vi "Test Binning.vi"(11 "Test Case In":refnum<class "Test.Camera.lvclass">) -> (0 "error out":errorcluster, 3 "Test Case Out":refnum<class "Test.Camera.lvclass">)   [LabVIEW 2020, in "Test.Camera.lvclass"]
uses:
  Test.Camera.lvclass
  C:/Program Files (x86)/National Instruments/LabVIEW 2020/vi.lib/Astemes/LUnit/Test Case.lvclass
  g_industrial_cam/Camera/Camera.lvclass/Camera.ctl
  <vilib>/Astemes/LUnit/Test Case.lvclass/Test Case.ctl
  c3e2611f-c54f-4219-a549-b8da21c7f085.vi
  c7776276-95e4-4134-9906-b61dd734a09f.vi
  e74630cf-9c8b-4a3c-8b50-f04e46fa7099.vi
  0aa1576c-e916-4ad0-9a97-64bd3e4eb69b.vi
  g_industrial_cam/Camera/GetSetBinning.vi
  <vilib>/Astemes/LUnit/Core/LUnit Test Case/Private/Append Pass Result.vi
  <vilib>/Astemes/LUnit/Core/LUnit Test Case/Private/Append Fail Result.vi
  0aa1576c-e916-4ad0-9a97-64bd3e4eb69b.vi/9c5d11cd-9439-4240-a1ee-d9baace9c924.vi
  <vilib>/Astemes/LUnit/Core/LUnit Test Case/Private/Run In UI.vi
  <vilib>/Utility/error.llb/Clear Errors.vi
  g_industrial_cam/Camera/Check Not Disconnected.vi
  <vilib>/Utility/error.llb/Error Cluster From Error Code.vi
  Test.Camera.lvclass/Test.Camera.ctl
  <vilib>/Astemes/LUnit/Test Case.lvclass
  g_industrial_cam/Camera/Camera.lvclass
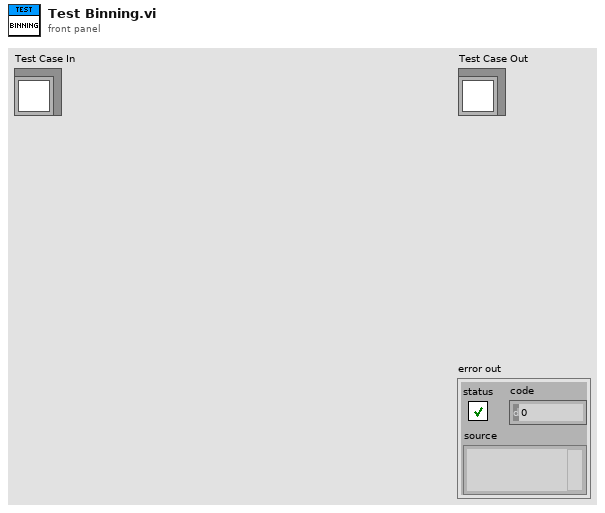
[diagram p1: front panel]
types:
  T1 = cluster{"dy Increment":i32, "dy Min":i32, "dy Max":i32, "dx Increment":i32, "dx Min":i32, "dx Max":i32, "dx":i32, "dy":i32, "Binning Avaliable":bool}
  T2 = cluster{"Alternative Value":i32, "Alternative Value":i32}
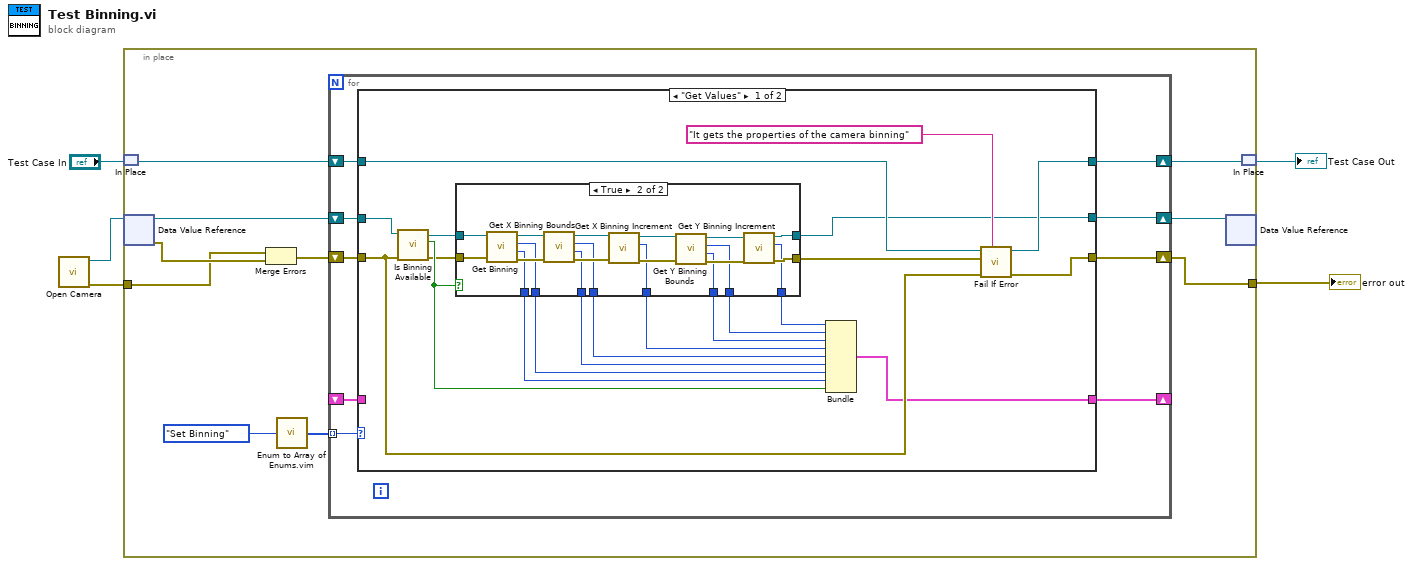
[diagram p0: block diagram]
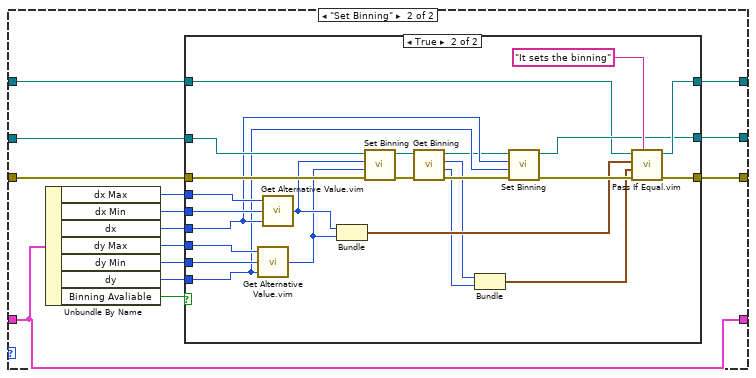
[diagram p3: hidden frame]
diagram:
  n1 = call "Open Camera.vi"() -> ("error out"=w5:errorcluster, "Camera"=w4:refnum<data-value>)  [unwired: 10 in]
  n2 = in-place {
    in-place-border: w5 -> [w9]
    in-place-border: [w8] -> w2
    n3 = in-place-match #1("Test Case In") -> (w10:refnum<class "Test.Camera.lvclass">)
    n4 = in-place-dvr #2(w4) -> (w14:refnum<class "Camera.lvclass">, w15:errorcluster)
    n5 = Merge Errors(w9, w15) -> (w13:errorcluster)
    n6 = call "Enum to Array of Enums.vim"("enum"=enum16{"Get Values", "Set Binning"}."Set Binning") -> ("array of enums"=w11:enum16{"Get Values", "Set Binning"}[])
    n7 = for {
      tunnel: w11 -> [w22] mode=indexing
      shift-right: [w21] -> w6
      shift-left: w14 -> [w24]
      shift-right: [w20] -> _
      shift-left: _ -> [w19]
      shift-right: [w17] -> w7
      shift-left: w10 -> [w18]
      shift-right: [w16] -> w8
      shift-left: w13 -> [w23]
      n8 = case shown="\"Get Values\"" w22 {
        tunnel: w24 -> [w40 w76]
        tunnel: w23 -> [w39 w77]
        tunnel: [w25 w69] -> w21
        tunnel: [w26 w78] -> w20
        tunnel: w19 -> [_ w78]
        tunnel: w18 -> [w44 w67]
        tunnel: [w43 w80] -> w17
        tunnel: [w41 w79] -> w16
        frame "Get Values" {
          n9 = call "Is Binning Available.vi"("error in (no error)"=w39, "Camera in"=w40) -> ("error out"=w37:errorcluster, "Binning Avaliable"=w38:bool, "Camera"=w36:refnum<class "Camera.lvclass">)  [unwired: 7 in]
          n10 = case shown="True" w38 {
            tunnel: w37 -> [w45 w66]
            tunnel: w36 -> [w46 w65]
            tunnel: [_ w59] -> w35
            tunnel: [_ w58] -> w34
            tunnel: [_ w57] -> w33
            tunnel: [_ w56] -> w32
            tunnel: [_ w55] -> w31
            tunnel: [_ w54] -> w30
            tunnel: [_ w53] -> w29
            tunnel: [w45 w52] -> w28
            tunnel: [_ w51] -> w27
            tunnel: [w46 w47] -> w25
            frame False {
            }
            frame True {
              n11 = call "Get Binning.vi"("error in (no error)"=w66, "Camera in"=w65) -> ("error out"=w64:errorcluster, "dy"=w59:i32, "dx"=w58:i32, "Camera"=w60:refnum<class "Camera.lvclass">)  [unwired: 6 in]
              n12 = call "Get X Binning Bounds.vi"("error in (no error)"=w64, "Camera in"=w60) -> ("error out"=w63:errorcluster, "dx Max"=w57:i32, "dx Min"=w56:i32, "Camera"=w50:refnum<class "Camera.lvclass">)  [unwired: 6 in]
              n13 = call "Get X Binning Increment.vi"("error in (no error)"=w63, "Camera in"=w50) -> ("error out"=w62:errorcluster, "dx Increment"=w55:i32, "Camera"=w49:refnum<class "Camera.lvclass">)  [unwired: 7 in]
              n14 = call "Get Y Binning Bounds.vi"("error in (no error)"=w62, "Camera in"=w49) -> ("error out"=w61:errorcluster, "dy Max"=w54:i32, "dy Min"=w53:i32, "Camera"=w48:refnum<class "Camera.lvclass">)  [unwired: 6 in]
              n15 = call "Get Y Binning Increment.vi"("error in (no error)"=w61, "Camera in"=w48) -> ("error out"=w52:errorcluster, "dy Increment"=w51:i32, "Camera"=w47:refnum<class "Camera.lvclass">)  [unwired: 7 in]
            }
          }
          n16 = Bundle("dy Increment"=w27, "dy Min"=w29, "dy Max"=w30, "dx Increment"=w31, "dx Min"=w32, "dx Max"=w33, "dx"=w34, "dy"=w35, "Binning Avaliable"=w38) -> (w26:T1)  [unwired: 1 in]
          n17 = call <vilib>:"Fail If Error.vi"("Description"="It gets the properties of the camera binning", "error in (no error)"=w39, "Assert error"=w28, "LUnit Test Case In"=w44) -> ("error out"=w41:errorcluster, "LUnit Test Case Out"=w43:refnum<class "Test.Camera.lvclass">)  [unwired: 6 in]
        }
        frame "Set Binning" {
          n18 = Unbundle By Name(w78) -> ("dx Max"=w75:i32, "dx Min"=w74:i32, "dx"=w73:i32, "dy Max"=w72:i32, "dy Min"=w71:i32, "dy"=w70:i32, "Binning Avaliable"=w68:bool)
          n19 = case shown="True" w68 {
            tunnel: [w83 w106] -> w80
            tunnel: [w81 w105] -> w79
            tunnel: w77 -> [w81 w103]
            tunnel: w76 -> [w82 w102]
            tunnel: w75 -> [_ w101]
            tunnel: w74 -> [_ w100]
            tunnel: w73 -> [_ w99]
            tunnel: w72 -> [_ w98]
            tunnel: w71 -> [_ w97]
            tunnel: w70 -> [_ w96]
            tunnel: [w82 w93] -> w69
            tunnel: w67 -> [w83 w84]
            frame False {
            }
            frame True {
              n20 = call "Get Alternative Value.vim"("Value"=w96, "Min"=w97, "Max"=w98) -> ("Alternative Value"=w91:i32)  [unwired: 1 in]
              n21 = call "Get Alternative Value.vim"("Value"=w99, "Min"=w100, "Max"=w101) -> ("Alternative Value"=w92:i32)  [unwired: 1 in]
              n22 = Bundle("Alternative Value"=w92, "Alternative Value"=w91) -> (w94:T2)  [unwired: 1 in]
              n23 = call "Set Binning.vi"("error in (no error)"=w103, "dy"=w91, "dx"=w92, "Camera in"=w102) -> ("error out"=w89:errorcluster, "Camera"=w90:refnum<class "Camera.lvclass">)  [unwired: 6 in]
              n24 = call "Get Binning.vi"("error in (no error)"=w89, "Camera in"=w90) -> ("error out"=w88:errorcluster, "dy"=w86:i32, "dx"=w85:i32, "Camera"=w87:refnum<class "Camera.lvclass">)  [unwired: 6 in]
              n25 = Bundle("dx"=w85, "dy"=w86) -> (w95:cluster{"dx":i32, "dy":i32})  [unwired: 1 in]
              n26 = call "Set Binning.vi"("error in (no error)"=w88, "dy"=w96, "dx"=w99, "Camera in"=w87) -> ("error out"=w107:errorcluster, "Camera"=w93:refnum<class "Camera.lvclass">)  [unwired: 6 in]
              n27 = call "Pass If Equal.vim"("Description"="It sets the binning", "error in (no error)"=w107, "Actual"=w95, "Expected"=w94, "LUnit Test Case In"=w84) -> ("error out"=w105:errorcluster, "LUnit Test Case Out"=w106:refnum<class "Test.Camera.lvclass">)  [unwired: 5 in]
            }
          }
        }
      }
    }
    n28 = in-place-dvr #2(w6) -> ()  [unwired: 2 out]
    n29 = in-place-match #1(w7) -> (→"Test Case Out":refnum<class "Test.Camera.lvclass">)
  }
  "error out" <- w2
